vi "BuildNetworkScanArray.vi"() -> ()   [LabVIEW 2018, in "MasterProgramSupportFunctions.lvlib"]
uses:
  MasterProgramSupportFunctions.lvlib
  TargetCluster.ctl
  TargetScanControlArray.ctl
  VI_tags.ctl
panel:
  in  "Target command Array":T1[](array[typedef]) {"target scan command"."target header"."action" items=["edit", "switch", "launch"]}
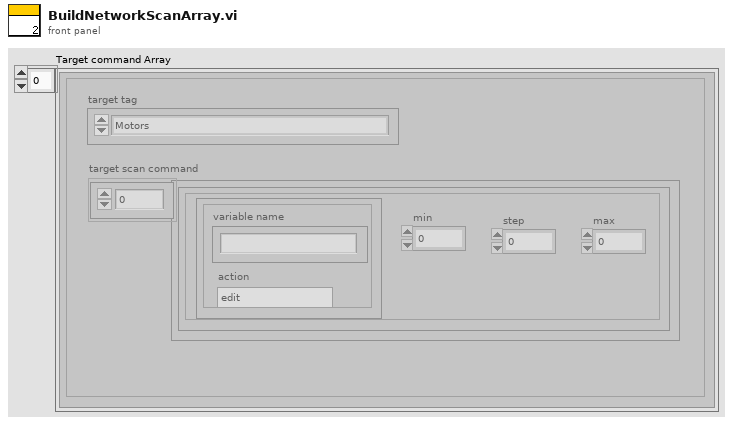
[diagram p1: front panel]
types:
  T1 = typedef "MasterProgramSupportFunctions.lvlib/TargetCluster.ctl" = cluster{"target scan command":T2, "target tag":T3}
  T2 = typedef "MasterProgramSupportFunctions.lvlib/TargetScanControlArray.ctl" = cluster{"min":dbl, "step":dbl, "max":dbl, "target header":cluster{"variable name":string, "action":u16}}[]
  T3 = typedef "MasterProgramSupportFunctions.lvlib/VI_tags.ctl" = enum16{"Motors", "Gage", "Tektro3107", "XimeaMainCamera", "ContinuousMainScan"}
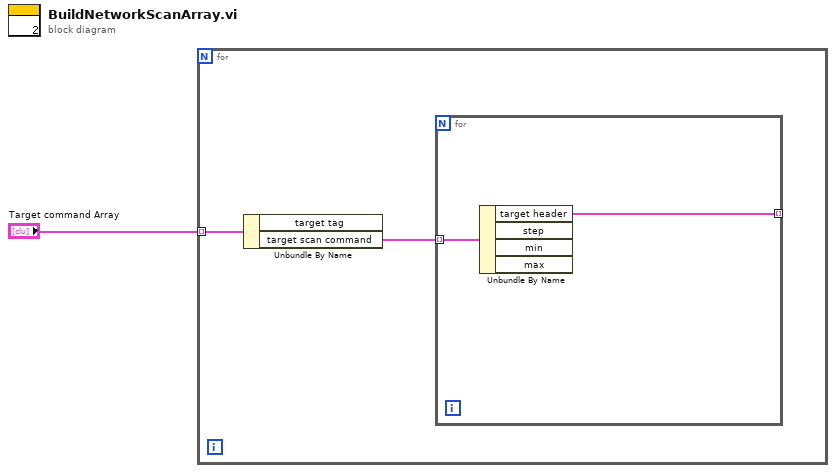
[diagram p0: block diagram]
diagram:
  n1 = for {
    tunnel: "Target command Array" -> [w3] mode=indexing
    n2 = Unbundle By Name(w3) -> ("target scan command"=w2:T2)  [unwired: 1 out]
    n3 = for {
      tunnel: w2 -> [w5] mode=indexing
      tunnel: [w4] -> _ mode=indexing
      n4 = Unbundle By Name(w5) -> ("target header"=w4:cluster{"variable name":string, "action":u16})  [unwired: 3 out]
    }
  }
